vi "Trapezoidal_Control_SubVI.vi"(2 "Current_Time":dbl, 3 "Inputs":T1) -> (0 "pSetProfile":dbl, 1 "vSetProfile":dbl)   [LabVIEW 2014]
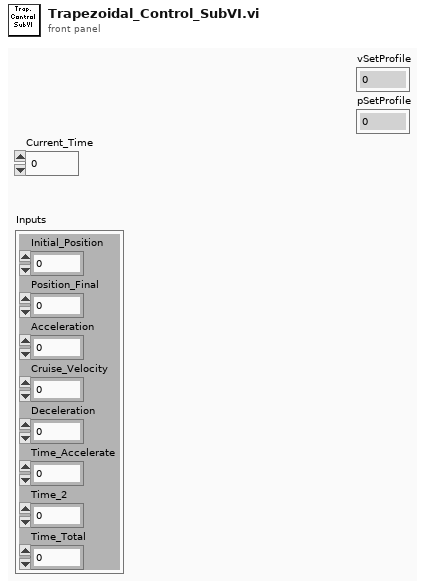
[diagram p1: front panel]
types:
  T1 = cluster{"Initial_Position":dbl, "Position_Final":dbl, "Acceleration":dbl, "Cruise_Velocity":dbl, "Deceleration":dbl, "Time_Accelerate":dbl, "Time_2":dbl, "Time_Total":dbl}
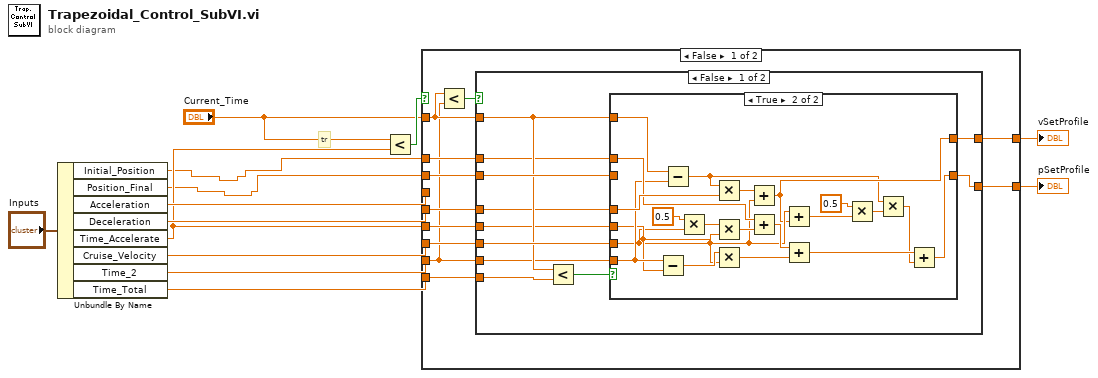
[diagram p0: block diagram]
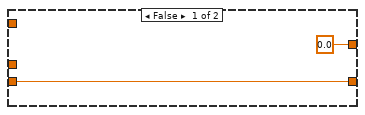
[diagram p2: hidden frame]
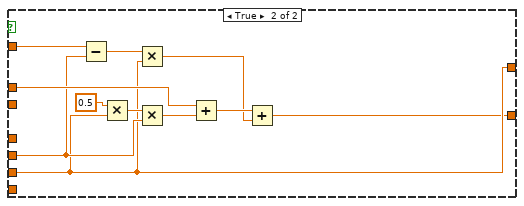
[diagram p3: hidden frame]
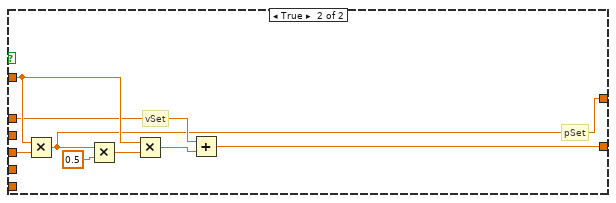
[diagram p4: hidden frame]
diagram:
  # "tr"
  n1 = Unbundle By Name("Inputs") -> ("Initial_Position"=w2:dbl, "Position_Final"=w1:dbl, "Acceleration"=w8:dbl, "Deceleration"=w7:dbl, "Time_Accelerate"=w6:dbl, "Cruise_Velocity"=w5:dbl, "Time_2"=w4:dbl, "Time_Total"=w3:dbl)
  n2 = Less?(x="Current_Time", y=w6) -> (x < y?=w13:bool)
  n3 = case shown="False" w13 {
    tunnel: w8 -> [_ w77]
    tunnel: "Current_Time" -> [w19 w74]
    tunnel: w2 -> [w21 w72]
    tunnel: [w18 w71] -> w11
    tunnel: [w22 w70] -> w12
    tunnel: w4 -> [w14 _]
    tunnel: w5 -> [w23 _]
    tunnel: w6 -> [w20 _]
    tunnel: w3 -> [w17 _]
    tunnel: w1 -> [w16 _]
    tunnel: w7 -> [w15 _]
    frame False {
      n4 = Less? ("Less? 2")(x=w19, y=w14) -> (x < y?=w24:bool)
      n5 = case "Case Structure 2" shown="False" w24 {
        tunnel: w23 -> [w30 w61]
        tunnel: [w33 w61] -> w22
        tunnel: w21 -> [w26 w69]
        tunnel: w20 -> [w25 w63]
        tunnel: w19 -> [w29 w64]
        tunnel: [w31 w59] -> w18
        tunnel: w17 -> [w34 _]
        tunnel: w16 -> [w32 _]
        tunnel: w15 -> [w27 _]
        tunnel: w14 -> [w28 _]
        frame False {
          n6 = Less? ("Less? 3")(x=w29, y=w34) -> (x < y?=w35:bool)
          n7 = case "Case Structure 3" shown="True" w35 {
            tunnel: [0.0 ("y 3") w45] -> w33
            tunnel: [w36 w38] -> w31
            tunnel: w32 -> [w36 _]
            tunnel: w30 -> [_ w46]
            tunnel: w29 -> [_ w52]
            tunnel: w28 -> [_ w48]
            tunnel: w27 -> [_ w51]
            tunnel: w26 -> [_ w49]
            tunnel: w25 -> [_ w47]
            frame False {
            }
            frame True {
              n8 = Subtract ("Subtract 3")(x=w48, y=w47) -> (x-y=w54:dbl)
              n9 = Subtract ("Subtract 4")(x=w52, y=w48) -> (x-y=w41:dbl)
              n10 = Multiply ("Multiply 7")(x=0.5 ("x 2"), y=w46) -> (x*y=w57:dbl)
              n11 = Multiply ("Multiply 10")(x=w41, y=w51) -> (x*y=w50:dbl)
              n12 = Multiply ("Multiply 8")(x=w57, y=w47) -> (x*y=w56:dbl)
              n13 = Multiply ("Multiply 9")(x=w54, y=w46) -> (x*y=w53:dbl)
              n14 = Add ("Add 6")(x=w50, y=w46) -> (x+y=w45:dbl)
              n15 = Add ("Add 4")(x=w49, y=w56) -> (x+y=w55:dbl)
              n16 = Add ("Add 7")(x=w46, y=w45) -> (x+y=w44:dbl)
              n17 = Add ("Add 5")(x=w55, y=w53) -> (x+y=w40:dbl)
              n18 = Multiply ("Multiply 11")(x=0.5 ("x 3"), y=w44) -> (x*y=w42:dbl)
              n19 = Multiply ("Multiply 12")(x=w41, y=w42) -> (x*y=w39:dbl)
              n20 = Add ("Add 8")(x=w40, y=w39) -> (x+y=w38:dbl)
            }
          }
        }
        frame True {
          n21 = Subtract ("Subtract 2")(x=w64, y=w63) -> (x-y=w62:dbl)
          n22 = Multiply ("Multiply 4")(x=0.5, y=w61) -> (x*y=w67:dbl)
          n23 = Multiply ("Multiply 6")(x=w62, y=w61) -> (x*y=w60:dbl)
          n24 = Multiply ("Multiply 5")(x=w67, y=w63) -> (x*y=w66:dbl)
          n25 = Add ("Add 2")(x=w69, y=w66) -> (x+y=w65:dbl)
          n26 = Add ("Add 3")(x=w65, y=w60) -> (x+y=w59:dbl)
        }
      }
    }
    frame True {
      # "pSet"
      # "vSet"
      n27 = Multiply(x=w74, y=w77) -> (x*y=w70:dbl)
      n28 = Multiply ("Multiply 2")(x=w70, y=0.5 ("y 2")) -> (x*y=w75:dbl)
      n29 = Multiply ("Multiply 3")(x=w74, y=w75) -> (x*y=w73:dbl)
      n30 = Add(x=w72, y=w73) -> (x+y=w71:dbl)
    }
  }
  "vSetProfile" <- w12
  "pSetProfile" <- w11
